vi "Interpolate 2D Scattered_Gn.vi"(0 "X(Tri) In":dbl[][](array[numeric]), 5 "Y(Tri) In":dbl[][](array[numeric]), 7 "Z(Tri) In":dbl[][](array[numeric]), 9 "gx in":dbl[][](array[numeric]), 11 "gy in":dbl[][](array[numeric]), 12 "Length":dbl[][](array[numeric])) -> (4 "X(Tri) Out":dbl[][](array[numeric]), 6 "Y(Tri) Out":dbl[][](array[numeric]), 8 "Z(Tri) Out":dbl[][](array[numeric]), 10 "gx out":dbl[][](array[numeric]), 14 "Gn":dbl[][](array[numeric]), 15 "gy out":dbl[][](array[numeric]))   [LabVIEW 2020, in "NI_AAL_Interpolation.lvlib"]
uses:
  <vilib>/gmath/NI_AAL_Interpolation.lvlib
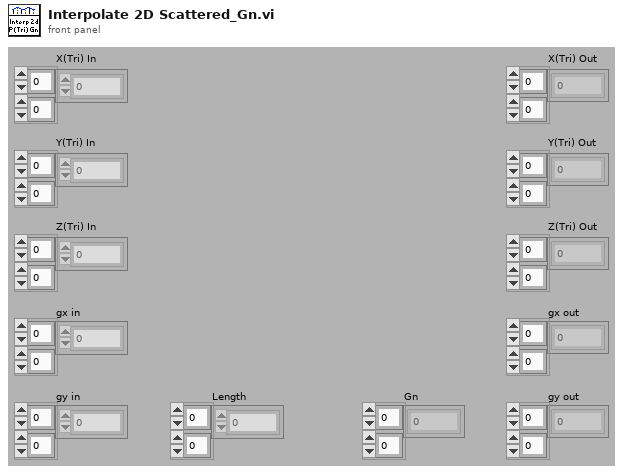
[diagram p1: front panel]
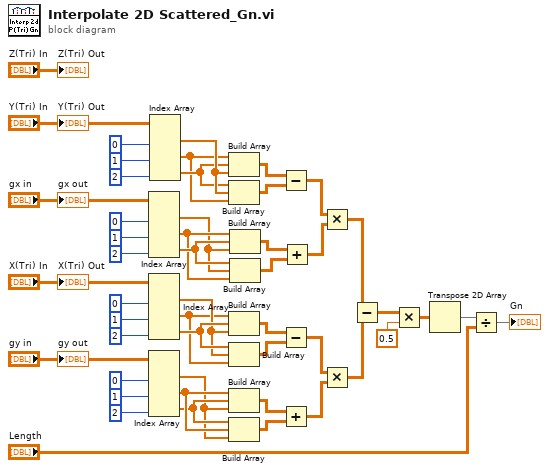
[diagram p0: block diagram]
diagram:
  n1 = Index Array(array="gx in", index (col) #1=0 ("disabled index (col)"), index (col) #2=1 ("index (col)"), index (col) #3=2 ("index (col)")) -> (element #1=w24:dbl[], element #2=w25:dbl[], element #3=w26:dbl[])  [unwired: 3 in]
  n2 = Index Array(array="X(Tri) In", index (col) #1=0 ("disabled index (col)"), index (col) #2=1 ("index (col)"), index (col) #3=2 ("index (col)")) -> (element #1=w31:dbl[], element #2=w30:dbl[], element #3=w32:dbl[])  [unwired: 3 in]
  n3 = Index Array(array="gy in", index (col) #1=0 ("disabled index (col)"), index (col) #2=1 ("index (col)"), index (col) #3=2 ("index (col)")) -> (element #1=w21:dbl[], element #2=w23:dbl[], element #3=w22:dbl[])  [unwired: 3 in]
  n4 = Index Array(array="Y(Tri) In", index (col) #1=0 ("disabled index (col)"), index (col) #2=1 ("index (col)"), index (col) #3=2 ("index (col)")) -> (element #1=w29:dbl[], element #2=w27:dbl[], element #3=w28:dbl[])  [unwired: 3 in]
  n5 = Build Array(w27, w28, w29) -> (w13:dbl[][])
  n6 = Build Array(w28, w29, w27) -> (w14:dbl[][])
  n7 = Build Array(w30, w32, w31) -> (w16:dbl[][])
  n8 = Build Array(w32, w31, w30) -> (w15:dbl[][])
  n9 = Build Array(w23, w22, w21) -> (w17:dbl[][])
  n10 = Build Array(w22, w23, w21) -> (w18:dbl[][])
  n11 = Build Array(w25, w26, w24) -> (w20:dbl[][])
  n12 = Build Array(w26, w24, w25) -> (w19:dbl[][])
  n13 = Subtract(x=w13, y=w14) -> (x-y=w12:dbl[][])
  n14 = Subtract(x=w16, y=w15) -> (x-y=w9:dbl[][])
  n15 = Add(x=w17, y=w18) -> (x+y=w10:dbl[][])
  n16 = Add(x=w20, y=w19) -> (x+y=w11:dbl[][])
  n17 = Multiply(x=w12, y=w11) -> (x*y=w8:dbl[][])
  n18 = Multiply(x=w9, y=w10) -> (x*y=w7:dbl[][])
  n19 = Subtract(x=w8, y=w7) -> (x-y=w6:dbl[][])
  n20 = Multiply(x=w6, y=0.5) -> (x*y=w4:dbl[][])
  n21 = Transpose 2D Array(2D array=w4) -> (transposed array=w3:dbl[][])
  n22 = Divide(x=w3, y="Length") -> (x/y=→"Gn":dbl[][])
  "X(Tri) Out" <- "X(Tri) In"
  "Y(Tri) Out" <- "Y(Tri) In"
  "Z(Tri) Out" <- "Z(Tri) In"
  "gx out" <- "gx in"
  "gy out" <- "gy in"
